vi "Split Lines.vi"(8 "error in (no error)":errorcluster, 10 "spreadsheet string":string, 11 "Setup File in":refnum<class "Setup File.lvclass">) -> (0 "error out":errorcluster, 2 "array":string[](array[string]), 3 "Setup File out":refnum<class "Setup File.lvclass">)   [LabVIEW 2018, in "Setup File.lvclass"]
uses:
  Setup File.lvclass
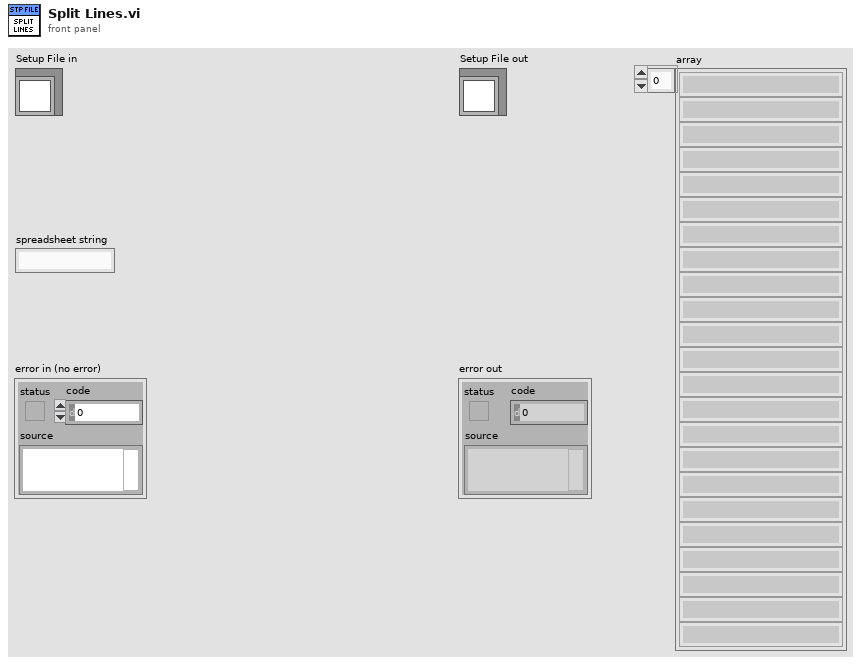
[diagram p1: front panel]
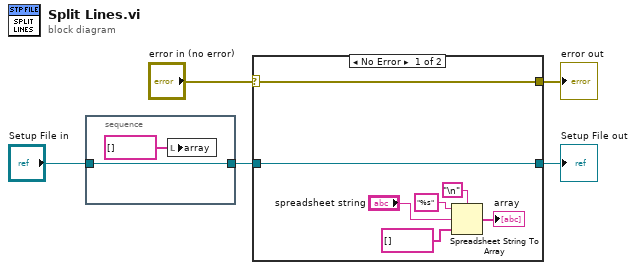
[diagram p0: block diagram]
diagram:
  n1 = stacked-sequence {
    tunnel: "Setup File in" -> [w6]
    tunnel: [w6] -> w3
    frame #0 {
      n2 = local write "array"(string[] []) -> ()
    }
  }
  n3 = case shown="No Error" "error in (no error)" {
    selector: "error in (no error)" -> [w13 w16]
    tunnel: [w13 w16] -> w1
    tunnel: [w14 w15] -> w2
    tunnel: w3 -> [w14 w15]
    frame No Error {
      n4 = Spreadsheet String To Array(delimiter (Tab)="\n", format string="%s", spreadsheet string="spreadsheet string", array type (2D Dbl)=string[] []) -> (array=→"array":string[])
    }
    frame Error {
    }
  }
  "error out" <- w1
  "Setup File out" <- w2
